vi "Autonomous Independent.vi"   [LabVIEW 2011]
doc: "This VI is called when autonomous begins, and will automatically be terminated when autonomous ends. You can carry out timed or sensor driven robot movement independently without needing to return to the caller."
uses:
  Robot Global Data.vi
types:
  T1 = typedef "WPI_MotorControlDeviceRef.ctl" = cluster{"DeviceStatus":errorcluster, "Type":enum16{"PWM", "CAN"}, "PWM":cluster{"Digital Module":T2, "PWM Channel":T3, "DeadBand":T4}, "CAN":cluster{"Device Number":u8, "Control Mode":T5, "Semaphore":T6, "Max Vout":dbl}, "Invert":bool, "TransformRef":T7, "InvTransformRef":T7}
  T2 = typedef "FPGA_TypedefDigitalModule.ctl" = enum16{"Digital Module 1", "Digital Module 2"}
  T3 = typedef "FPGA_DIOPWMChannel.ctl" = enum8{"PWM 1", "PWM 2", "PWM 3", "PWM 4", "PWM 5", "PWM 6", "PWM 7", "PWM 8", "PWM 9", "PWM 10", "Invalid"}
  T4 = typedef "WPI_PWMDeadband.ctl" = cluster{"Name":string, "maxPositivePwm":i32, "minPositivePwm":i32, "centerPwm":i32, "maxNegativePwm":i32, "minNegativePwm":i32, "angularRange":u16}
  T5 = typedef "WPI_CANJaguar_ControlMode.ctl" = enum8{"Percent VBus", "Current", "Speed", "Position", "Voltage"}
  T6 = typedef "Semaphore RefNum" = refnum<k1>
  T7 = typedef "WPI_PWMTransform_ConPane.ctl" = refnum<vi>
  T8 = typedef "WPI_ServoDeviceRef.ctl" = cluster{"DeviceStatus":errorcluster, "Digital Module":T2, "PWM Channel":T3, "DeadBand":T4}
  T9 = typedef "WPI_EncoderDevRef.ctl" = cluster{"DevStatus":errorcluster, "EncoderIndex":T10, "CounterIndex":T11, "DistancePerCount":dbl, "Decoding Type":T12}
  T10 = typedef "FPGA_EncoderIdx.ctl" = enum8{"Enc 0", "Enc 1", "Enc 2", "Enc 3", "Invalid"}
  T11 = typedef "FPGA_CounterCtrSystemIndex.ctl" = enum8{"Ctr 0", "Ctr 1", "Ctr 2", "Ctr 3", "Ctr 4", "Ctr 5", "Ctr 6", "Ctr 7", "Invalid"}
  T12 = typedef "WPI_EncoderType.ctl" = enum16{"1x", "2x", "4x"}
  T13 = typedef "WPI_GyroDevRef.ctl" = cluster{"DevStatus":errorcluster, "Analog Module":T14, "Analog Channel":T15, "Offset":dbl, "Gain (VoltsPerDegree/Second)":dbl}
  T14 = typedef "FPGA_TypedefAnalogModule.ctl" = enum16{"Analog Module 1", "Analog Module 2"}
  T15 = typedef "FPGA_AIChannel.ctl" = enum8{"AI 1", "AI 2", "AI 3", "AI 4", "AI 5", "AI 6", "AI 7", "AI 8", "Invalid"}
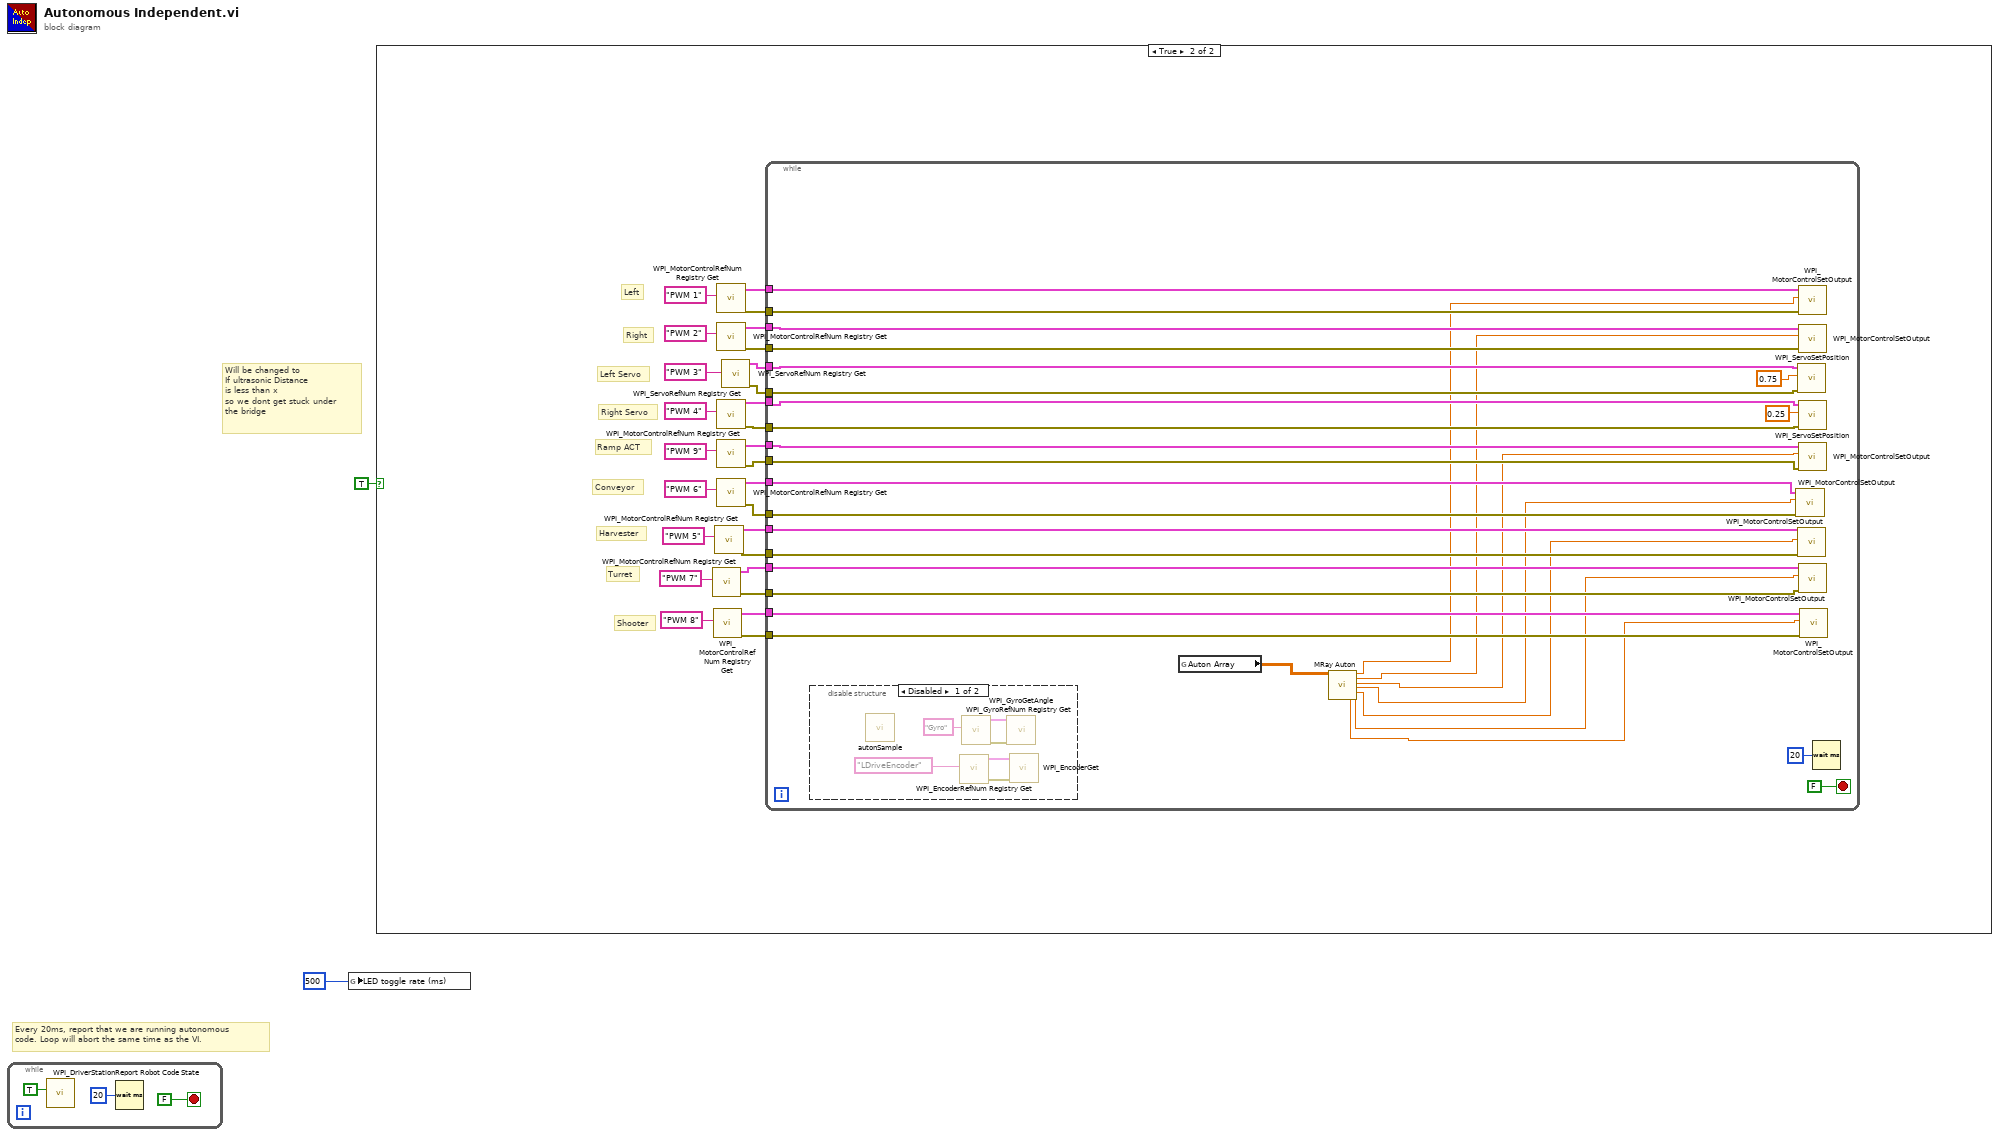
[diagram p0: block diagram]
diagram:
  # "Will be changed to\nIf ultrasonic Distance \nis less than x\nso we dont get stuck under \nthe bridge"
  # "Every 20ms, report that we are running autonomous\ncode. Loop will abort the same time as the VI."
  n1 = while {
    stop <- FALSE stop-if-true
    n2 = call <vilib>:"WPI_DriverStationReport Robot Code State.vi"("Autonomous"=TRUE) -> ()  [unwired: 10 in, 1 out]
    n3 = Wait (ms)(milliseconds to wait=u32 20) -> ()  [unwired: 1 out]
  }
  n4 = global write "Robot Global Data.vi" "LED toggle rate (ms)"(u32 500 ("LED ms toggle rate")) -> ()
  n5 = case shown="True" TRUE {
    frame False {
    }
    frame True {
      # "Shooter"
      # "Turret"
      # "Conveyor"
      # "Harvester"
      # "Ramp ACT"
      # "Right Servo"
      # "Left Servo"
      # "Right"
      # "Left"
      n6 = call <vilib>:"WPI_MotorControlRefNum Registry Get.vi"("refnum name"="PWM 7") -> ("error out"=w13:errorcluster, "MotorControlDevRef"=w14:T1)  [unwired: 9 in]
      n7 = call <vilib>:"WPI_MotorControlRefNum Registry Get.vi"("refnum name"="PWM 8") -> ("error out"=w11:errorcluster, "MotorControlDevRef"=w12:T1)  [unwired: 9 in]
      n8 = call <vilib>:"WPI_MotorControlRefNum Registry Get.vi"("refnum name"="PWM 5") -> ("error out"=w15:errorcluster, "MotorControlDevRef"=w16:T1)  [unwired: 9 in]
      n9 = call <vilib>:"WPI_MotorControlRefNum Registry Get.vi"("refnum name"="PWM 1") -> ("error out"=w6:errorcluster, "MotorControlDevRef"=w28:T1)  [unwired: 9 in]
      n10 = call <vilib>:"WPI_MotorControlRefNum Registry Get.vi"("refnum name"="PWM 2") -> ("error out"=w7:errorcluster, "MotorControlDevRef"=w27:T1)  [unwired: 9 in]
      n11 = call <vilib>:"WPI_ServoRefNum Registry Get.vi"("refnum name"="PWM 4") -> ("error out"=w9:errorcluster, "ServoDeviceRef"=w26:T8)  [unwired: 9 in]
      n12 = call <vilib>:"WPI_MotorControlRefNum Registry Get.vi"("refnum name"="PWM 9") -> ("error out"=w10:errorcluster, "MotorControlDevRef"=w25:T1)  [unwired: 9 in]
      n13 = call <vilib>:"WPI_MotorControlRefNum Registry Get.vi"("refnum name"="PWM 6") -> ("error out"=w20:errorcluster, "MotorControlDevRef"=w21:T1)  [unwired: 9 in]
      n14 = call <vilib>:"WPI_ServoRefNum Registry Get.vi"("refnum name"="PWM 3") -> ("error out"=w8:errorcluster, "ServoDeviceRef"=w23:T8)  [unwired: 9 in]
      n15 = while {
        tunnel: w28 -> [w60]
        tunnel: w27 -> [w59]
        tunnel: w23 -> [w54]
        tunnel: w26 -> [w55]
        tunnel: w25 -> [w58]
        tunnel: w21 -> [w53]
        tunnel: w20 -> [w52]
        tunnel: w16 -> [w51]
        tunnel: w15 -> [w50]
        tunnel: w14 -> [w49]
        tunnel: w13 -> [w48]
        tunnel: w12 -> [w47]
        tunnel: w11 -> [w46]
        tunnel: w10 -> [w45]
        tunnel: w9 -> [w44]
        tunnel: w8 -> [w43]
        tunnel: w7 -> [w42]
        tunnel: w6 -> [w41]
        stop <- FALSE stop-if-true
        n16 = disable-structure shown="Disabled" {
          frame Disabled {
            n17 = call "autonSample.vi"() -> ()  [unwired: 9 in, 7 out]
            n18 = call <vilib>:"WPI_EncoderRefNum Registry Get.vi"("refnum name"="LDriveEncoder") -> ("error out"=w66:errorcluster, "EncoderDevRef"=w67:T9)  [unwired: 9 in]
            n19 = call <vilib>:"WPI_GyroRefNum Registry Get.vi"("refnum name"="Gyro") -> ("error out"=w64:errorcluster, "GyroDevRef"=w65:T13)  [unwired: 9 in]
            n20 = call <vilib>:"WPI_GyroGetAngle.vi"("error in (no error)"=w64, "GyroDevRef"=w65) -> ()  [unwired: 6 in, 4 out]
            n21 = call <vilib>:"WPI_EncoderGet.vi"("error in (no error)"=w66, "EncoderDevRef"=w67) -> ()  [unwired: 4 in, 6 out]
          }
          frame Enabled {
          }
        }
        n22 = global read "Robot Global Data.vi" "Auton Array"() -> (w40:dbl[][])
        n23 = call "MRay Auton.vi"("Auton Array"=w40) -> ("Shooter"=w33:dbl, "Left Drive"=w39:dbl, "Right Drive"=w38:dbl, "Ramp ACT motor"=w37:dbl, "Conveyor"=w36:dbl, "Harvester"=w35:dbl, "Turret Rotation"=w34:dbl)  [unwired: 12 in]
        n24 = call <vilib>:"WPI_MotorControlSetOutput.vi"("error in (no error)"=w52, "Output"=w36, "MotorControlDevRef"=w53) -> ()  [unwired: 7 in, 2 out]
        n25 = call <vilib>:"WPI_ServoSetPosition.vi"("error in (no error)"=w43, "Position"=0.75 ("Output"), "ServoDeviceRef"=w54) -> ()  [unwired: 7 in, 2 out]
        n26 = call <vilib>:"WPI_MotorControlSetOutput.vi"("error in (no error)"=w50, "Output"=w35, "MotorControlDevRef"=w51) -> ()  [unwired: 7 in, 2 out]
        n27 = call <vilib>:"WPI_MotorControlSetOutput.vi"("error in (no error)"=w41, "Output"=w39, "MotorControlDevRef"=w60) -> ()  [unwired: 7 in, 2 out]
        n28 = call <vilib>:"WPI_MotorControlSetOutput.vi"("error in (no error)"=w42, "Output"=w38, "MotorControlDevRef"=w59) -> ()  [unwired: 7 in, 2 out]
        n29 = call <vilib>:"WPI_ServoSetPosition.vi"("error in (no error)"=w44, "Position"=0.25 ("Output"), "ServoDeviceRef"=w55) -> ()  [unwired: 7 in, 2 out]
        n30 = call <vilib>:"WPI_MotorControlSetOutput.vi"("error in (no error)"=w45, "Output"=w37, "MotorControlDevRef"=w58) -> ()  [unwired: 7 in, 2 out]
        n31 = call <vilib>:"WPI_MotorControlSetOutput.vi"("error in (no error)"=w48, "Output"=w34, "MotorControlDevRef"=w49) -> ()  [unwired: 7 in, 2 out]
        n32 = call <vilib>:"WPI_MotorControlSetOutput.vi"("error in (no error)"=w46, "Output"=w33, "MotorControlDevRef"=w47) -> ()  [unwired: 7 in, 2 out]
        n33 = Wait (ms)(milliseconds to wait=u32 20) -> ()  [unwired: 1 out]
      }
    }
  }
